vi "Trans_RT.vi"() -> ()   [LabVIEW 2016]
uses:
  PRIME Lab 2017b/Control/PRIME Control 2017b/Controls/GP307 cluster.ctl
  <vilib>/FPGAPlugInAG/cRIO-9067/niLvFpga_Open_cRIO-9067.vi
  <vilib>/Utility/error.llb/Error Cluster From Error Code.vi
  <vilib>/rvi/errors/niLvFpgaAdjustHostInterfaceError.vi
  <vilib>/functionblocks/Control/PID/PID.vi
  <vilib>/rvi/interface/nirviOpenFPGA/nirviOpenFPGA.xnode
  Builds/cRIOs/Trans-cRIO/FPGA/PRIMEControl2017_FPGA-Trans_FPGATrans_z3cvJGH+foY.lvbitx
  Trans_FPGA.vi
  <vilib>/rvi/interface/nirviReadWriteControl/nirviReadWriteControl.xnode
  <vilib>/functionblocks/FB Core/FB Core.xnode
  <vilib>/functionblocks/FB Property/FB Overlay DBL.ctl
  <vilib>/functionblocks/NI_FunctionBlock Libraries.lvlib
  <vilib>/NI_Real-Time Target Support.lvlib
  NiFpgaLv.dll
panel:
  in  "Tab Control":T1(tab)
  in  "derivative time (Td, min) -analyzer":dbl=0.05
  in  "integral time (Ti, min) -analyzer":dbl=0.01
  in  "proportional gain (Kc) -analyzer":dbl=25.0
  out "Analyzer mag command string":string
  out "analyzer field read":dbl
  out "Analyzer mag command":u8[](array[numeric])
  out "Analyzer mag field read":u8[](array[numeric])
  out "Analyzer mag field set":dbl
  in  "output high - analyzer":dbl=300.0
  in  "output low - analyzer":dbl
  out "Switch mag field set":dbl
  out "Switch mag field read":u8[](array[numeric])
  out "switch mag field read":dbl
  out "Switch mag command":u8[](array[numeric])
  in  "derivative time (Td, min) - switch":dbl=0.01
  in  "integral time (Ti, min) - switch":dbl=0.01
  in  "proportional gain (Kc) - switch":dbl=10.0
  out "Switch mag command string":string
  in  "output high - switch":dbl=250.0
  in  "output low - switch":dbl
  out "ExB mag command":u8[](array[numeric])
  out "EXB mag current set":dbl
  out "ExB mag command string":string
  out "Switch Mag addr command":u8[](array[numeric])
  out "Switch Mag ps trig":u8[](array[numeric])
  out "Steerer X+":dbl
  out "Steerer X-":dbl
  out "Steerer Y+":dbl
  out "Steerer Y-":dbl
  out "ExB +":dbl
  out "ExB -":dbl
  out "X+ V":fxp<+/-,26,5> format="%.23g"
  out "X+ I":fxp<+/-,26,5> format="%_4g"
  out "X- V":fxp<+/-,26,5> format="%_4g"
  out "X- I":fxp<+/-,26,5> format="%_4g"
  out "Y+ V":fxp<+/-,26,5> format="%_4g"
  out "Y+ I":fxp<+/-,26,5> format="%_4g"
  out "Y- V":fxp<+/-,26,5> format="%_4g"
  out "Y- I":fxp<+/-,26,5> format="%_4g"
  out "ExB+ V":fxp<+/-,26,5> format="%_4g"
  out "ExB+ I":fxp<+/-,26,5> format="%_4g"
  out "ExB- V":fxp<+/-,26,5> format="%_4g"
  out "ExB- I":fxp<+/-,26,5> format="%_4g"
  in  "Ion gauge cluster control":T2
  out "Analyze image vac gauge cluster":T3
  out "Switch object vac gauge cluster":T3
  out "Convectron 4":u8[](array[numeric])
  out "Ion gauge 4":u8[](array[numeric])
  out "Convectron 3":u8[](array[numeric])
  out "Ion gauge 3":u8[](array[numeric])
  out "Convectron 2":u8[](array[numeric])
  out "Ion gauge 2":u8[](array[numeric])
  out "Convectron 1":u8[](array[numeric])
  out "Ion gauge 1":u8[](array[numeric])
  out "Readback loop error":errorcluster
  out "Vacuum loop error":errorcluster
  out "Control Loop error":errorcluster
  out "ExB error":errorcluster
  out "Switch Magnet error":errorcluster
  out "Analyzer Magnet error":errorcluster
  out "Trans RT Error":errorcluster
  out "Trans FPGA error":errorcluster
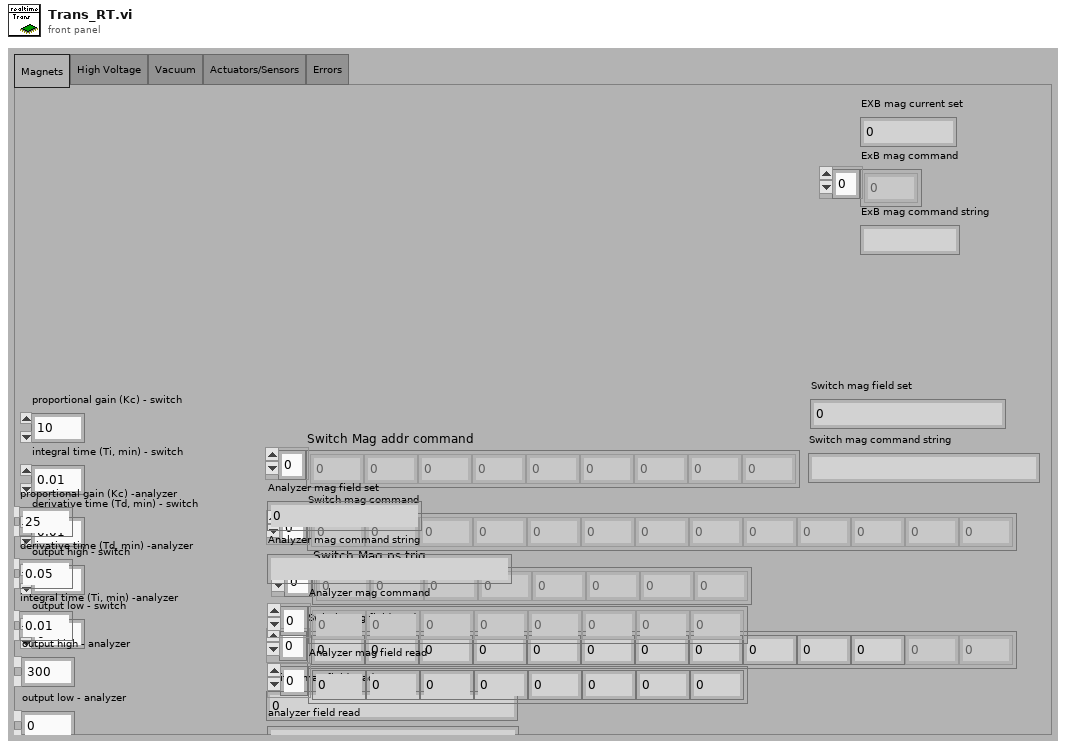
[diagram p1: front panel]
types:
  T1 = enum32{"Magnets", "High Voltage", "Vacuum", "Actuators/Sensors", "Errors"}
  T2 = typedef "GP307 cluster.ctl" = cluster{"Ion gauge 1":string, "Convectron  Gauge 1 ":string, "Ion Gauge 2":string, "Convectrom Gauge 2":string}
  T3 = cluster{"Ion gauge 1":string, "Convectron  Gauge 1 ":string, "Ion Gauge 2":string, "Convectrom Gauge 2":string}
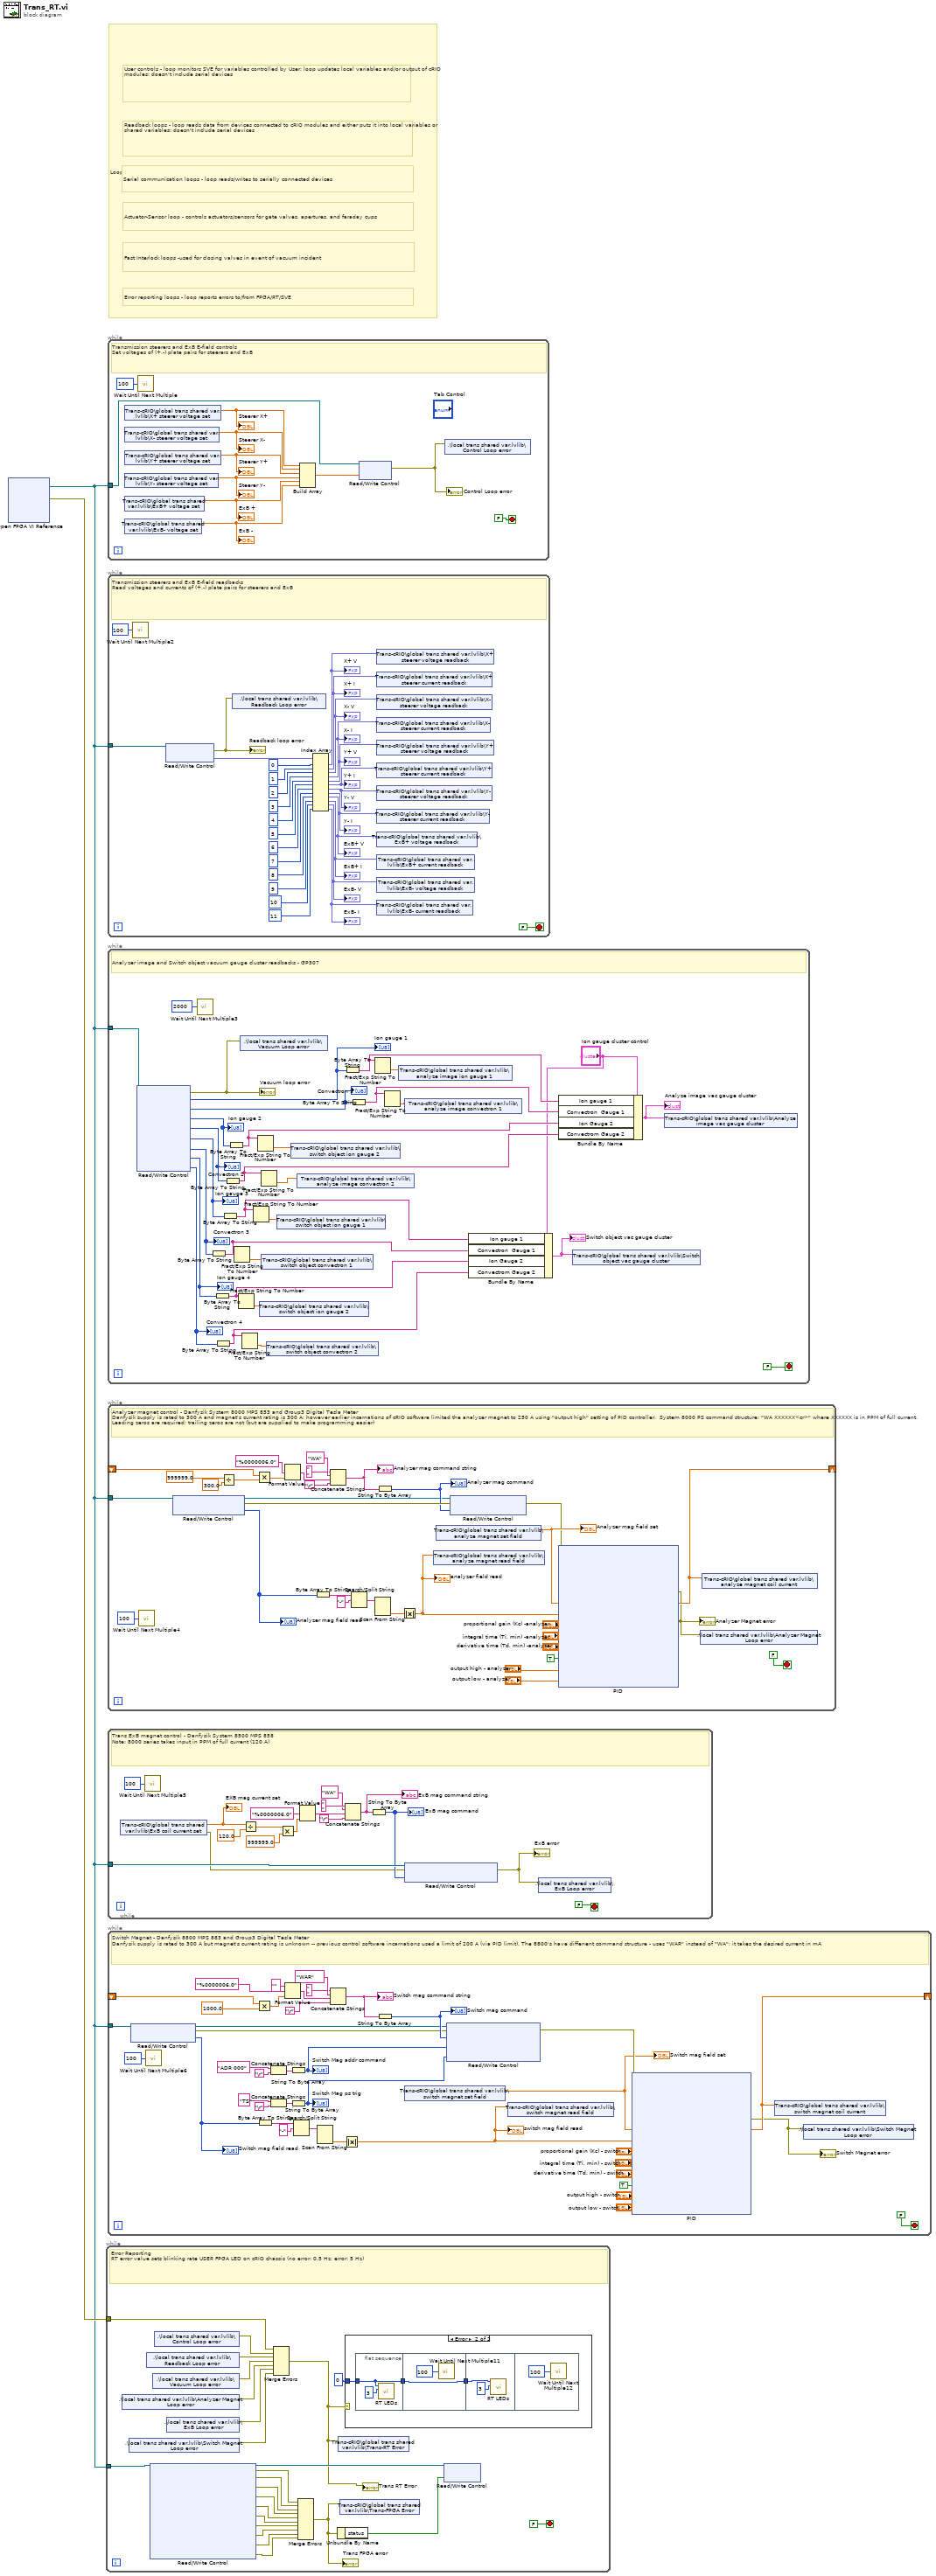
[diagram p0: block diagram]
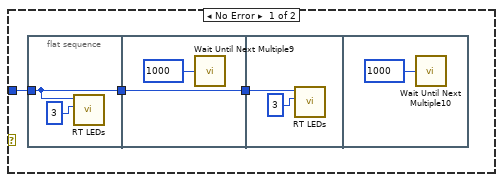
[diagram p2: hidden frame]
diagram:
  # "Serial communication loops - loop reads/writes to serially connected devices"
  # "Actuator-Sensor loop - controls actuators/sensors for gate valves, apertures, and faraday cups"
  # "Fast Interlock loops -used for closing valves in event of vacuum incident"
  # "Error reporting loops - loop reports errors to/from FPGA/RT/SVE"
  # "Readback loops - loop reads data from devices connected to cRIO modules and either puts it into local variables or shared variables; doesn't include serial devices"
  # "User controls - loop monitors SVE for variables controlled by User; loop updates local variables and/or output of cRIO modules; doesn't include serial devices"
  # "Loop legend - loops are color coded by responsibility"
  n1 = xnode "Open FPGA VI Reference"() -> ("FPGA VI Reference Out"=w1:refnum<k20>, "error out"=w2:errorcluster)  [unwired: 2 in]
  n2 = while {
    tunnel: w1 -> [w25]
    tunnel: w2 -> [w4]
    stop <- FALSE stop-if-true
    # "Error Reporting\nRT error value sets blinking rate USER FPGA LED on cRIO chassis (no error: 0.5 Hz; error: 5 Hz)"
    n3 = shared-variable ".\\local trans shared var.lvlib\\Analyzer Magnet Loop error"() -> (w10:errorcluster)  [unwired: 1 in, 1 out]
    n4 = shared-variable ".\\local trans shared var.lvlib\\Switch Magnet Loop error"() -> (w12:errorcluster)  [unwired: 1 in, 1 out]
    n5 = shared-variable ".\\local trans shared var.lvlib\\Readback Loop error"() -> (w8:errorcluster)  [unwired: 1 in, 1 out]
    n6 = xnode "Read/Write Control"("FPGA VI Reference In"=w25) -> ("FPGA VI Reference Out"=w24:refnum<k20>, "error out"=w13:errorcluster, "9205 error"=w23:errorcluster, "9264 error"=w22:errorcluster, "Analyzer PS error"=w21:errorcluster, "ExB PS error"=w20:errorcluster, "Switch PS error"=w19:errorcluster, "Analyzer Hall Probe error"=w18:errorcluster, "Switch Hall Probe error"=w17:errorcluster, "Analyze Image Vacuum Error"=w16:errorcluster, "Switch Object Vacuum Error"=w15:errorcluster)  [unwired: 1 in]
    n7 = shared-variable ".\\local trans shared var.lvlib\\Vacuum Loop error"() -> (w9:errorcluster)  [unwired: 1 in, 1 out]
    n8 = shared-variable ".\\local trans shared var.lvlib\\Control Loop error"() -> (w7:errorcluster)  [unwired: 1 in, 1 out]
    n9 = shared-variable ".\\local trans shared var.lvlib\\ExB Loop error"() -> (w11:errorcluster)  [unwired: 1 in, 1 out]
    n10 = Merge Errors(w4, w7, w8, w9, w10, w11, w12) -> (w3:errorcluster)
    "Trans RT Error" <- w3
    n11 = Merge Errors(w13, w23, w22, w21, w20, w19, w18, w17, w16, w15) -> (w6:errorcluster)
    "Trans FPGA error" <- w6
    n12 = Unbundle By Name(w6) -> ("status"=w26:bool)
    n13 = shared-variable "Trans-cRIO\\global trans shared var.lvlib\\Trans-RT Error"(w3) -> ()  [unwired: 1 in, 1 out]
    n14 = shared-variable "Trans-cRIO\\global trans shared var.lvlib\\Trans-FPGA Error"(w6) -> ()  [unwired: 1 in, 1 out]
    n15 = case shown="Error" w3 {
      tunnel: 0 -> [w29 w37]
      frame No Error {
        n16 = flat-sequence {
          tunnel: w29 -> [w30]
          tunnel: [w30] -> w27
          tunnel: [w32] -> w28
          tunnel: w27 -> [w32]
          tunnel: w28 -> [w34]
          frame #0 {
            n17 = call <vilib>:"RT LEDs.vi"("State"=3, "LED Num"=w30) -> ()  [unwired: 4 in, 2 out]
          }
          frame #1 {
            n18 = call "Wait Until Next Multiple9"("Count(mSec)"=u16 1000) -> ()  [unwired: 1 out]
          }
          frame #2 {
            n19 = call <vilib>:"RT LEDs.vi"("State"=3, "LED Num"=w34) -> ()  [unwired: 4 in, 2 out]
          }
          frame #3 {
            n20 = call "Wait Until Next Multiple10"("Count(mSec)"=u16 1000) -> ()  [unwired: 1 out]
          }
        }
      }
      frame Error {
        n21 = flat-sequence {
          tunnel: [w40] -> w39
          tunnel: w37 -> [w40]
          tunnel: w39 -> [w42]
          tunnel: [w42] -> w38
          tunnel: w38 -> [w44]
          frame #0 {
            n22 = call <vilib>:"RT LEDs.vi"("State"=3, "LED Num"=w40) -> ()  [unwired: 4 in, 2 out]
          }
          frame #1 {
            n23 = call "Wait Until Next Multiple11"("Count(mSec)"=u16 100) -> ()  [unwired: 1 out]
          }
          frame #2 {
            n24 = call <vilib>:"RT LEDs.vi"("State"=3, "LED Num"=w44) -> ()  [unwired: 4 in, 2 out]
          }
          frame #3 {
            n25 = call "Wait Until Next Multiple12"("Count(mSec)"=u16 100) -> ()  [unwired: 1 out]
          }
        }
      }
    }
    n26 = xnode "Read/Write Control"("FPGA VI Reference In"=w24, "RT error"=w26) -> ()  [unwired: 1 in, 2 out]
  }
  n27 = while {
    tunnel: w1 -> [w48]
    stop <- FALSE stop-if-true
    # "Transmission steerers and ExB E-field controls\nSet voltages of (+,-) plate pairs for steerers and ExB"
    n28 = shared-variable "Trans-cRIO\\global trans shared var.lvlib\\X+ steerer voltage set"() -> (w50:dbl)  [unwired: 1 in, 1 out]
    "Steerer X+" <- w50
    n29 = shared-variable "Trans-cRIO\\global trans shared var.lvlib\\X- steerer voltage set"() -> (w51:dbl)  [unwired: 1 in, 1 out]
    "Steerer X-" <- w51
    n30 = shared-variable "Trans-cRIO\\global trans shared var.lvlib\\Y+ steerer voltage set"() -> (w52:dbl)  [unwired: 1 in, 1 out]
    "Steerer Y+" <- w52
    n31 = shared-variable "Trans-cRIO\\global trans shared var.lvlib\\Y- steerer voltage set"() -> (w53:dbl)  [unwired: 1 in, 1 out]
    "Steerer Y-" <- w53
    n32 = shared-variable "Trans-cRIO\\global trans shared var.lvlib\\ExB+ voltage set"() -> (w54:dbl)  [unwired: 1 in, 1 out]
    "ExB +" <- w54
    n33 = shared-variable "Trans-cRIO\\global trans shared var.lvlib\\ExB- voltage set"() -> (w55:dbl)  [unwired: 1 in, 1 out]
    "ExB -" <- w55
    n34 = call "Wait Until Next Multiple"("Count(mSec)"=u32 100 ("millisecond multiple")) -> ()  [unwired: 1 out]
    n35 = Build Array(w50, w51, w52, w53, w54, w55) -> (w57:dbl[])
    n36 = xnode "Read/Write Control"("FPGA VI Reference In"=w48, "HV Set"=w57) -> ("error out"=w49:errorcluster)  [unwired: 1 in, 1 out]
    "Control Loop error" <- w49
    n37 = shared-variable ".\\local trans shared var.lvlib\\Control Loop error"(w49) -> ()  [unwired: 1 in, 1 out]
  }
  n38 = while {
    tunnel: w1 -> [w60]
    stop <- FALSE stop-if-true
    # "Transmission steerers and ExB E-field readbacks\nRead voltages and currents of (+,-) plate pairs for steerers and ExB"
    n39 = call "Wait Until Next Multiple2"("Count(mSec)"=u32 100 ("millisecond multiple")) -> ()  [unwired: 1 out]
    n40 = xnode "Read/Write Control"("FPGA VI Reference In"=w60) -> ("error out"=w59:errorcluster, "HV monitor"=w86:fxp<+/-,26,5>[])  [unwired: 1 in, 1 out]
    "Readback loop error" <- w59
    n41 = shared-variable ".\\local trans shared var.lvlib\\Readback Loop error"(w59) -> ()  [unwired: 1 in, 1 out]
    n42 = Index Array(array=w86, index #1=0 ("index"), index #2=1 ("index"), index #3=2 ("index"), index #4=3 ("index"), index #5=4 ("index"), index #6=5 ("index"), index #7=6 ("index"), index #8=7 ("index"), index #9=8 ("index"), index #10=9 ("index"), index #11=10 ("index"), index #12=11 ("index")) -> (element #1=w75:fxp<+/-,26,5>, element #2=w77:fxp<+/-,26,5>, element #3=w76:fxp<+/-,26,5>, element #4=w74:fxp<+/-,26,5>, element #5=w78:fxp<+/-,26,5>, element #6=w80:fxp<+/-,26,5>, element #7=w79:fxp<+/-,26,5>, element #8=w81:fxp<+/-,26,5>, element #9=w82:fxp<+/-,26,5>, element #10=w84:fxp<+/-,26,5>, element #11=w83:fxp<+/-,26,5>, element #12=w85:fxp<+/-,26,5>)
    "X+ V" <- w75
    "X+ I" <- w77
    "X- V" <- w76
    "X- I" <- w74
    "Y+ V" <- w78
    "Y+ I" <- w80
    "Y- V" <- w79
    "Y- I" <- w81
    "ExB+ V" <- w82
    "ExB+ I" <- w84
    "ExB- V" <- w83
    "ExB- I" <- w85
    n43 = shared-variable "Trans-cRIO\\global trans shared var.lvlib\\X+ steerer voltage readback"(w75) -> ()  [unwired: 1 in, 1 out]
    n44 = shared-variable "Trans-cRIO\\global trans shared var.lvlib\\X+ steerer current readback"(w77) -> ()  [unwired: 1 in, 1 out]
    n45 = shared-variable "Trans-cRIO\\global trans shared var.lvlib\\X- steerer voltage readback"(w76) -> ()  [unwired: 1 in, 1 out]
    n46 = shared-variable "Trans-cRIO\\global trans shared var.lvlib\\X- steerer current readback"(w74) -> ()  [unwired: 1 in, 1 out]
    n47 = shared-variable "Trans-cRIO\\global trans shared var.lvlib\\Y+ steerer voltage readback"(w78) -> ()  [unwired: 1 in, 1 out]
    n48 = shared-variable "Trans-cRIO\\global trans shared var.lvlib\\Y+ steerer current readback"(w80) -> ()  [unwired: 1 in, 1 out]
    n49 = shared-variable "Trans-cRIO\\global trans shared var.lvlib\\Y- steerer voltage readback"(w79) -> ()  [unwired: 1 in, 1 out]
    n50 = shared-variable "Trans-cRIO\\global trans shared var.lvlib\\Y- steerer current readback"(w81) -> ()  [unwired: 1 in, 1 out]
    n51 = shared-variable "Trans-cRIO\\global trans shared var.lvlib\\ExB+ voltage readback"(w82) -> ()  [unwired: 1 in, 1 out]
    n52 = shared-variable "Trans-cRIO\\global trans shared var.lvlib\\ExB+ current readback"(w84) -> ()  [unwired: 1 in, 1 out]
    n53 = shared-variable "Trans-cRIO\\global trans shared var.lvlib\\ExB- voltage readback"(w83) -> ()  [unwired: 1 in, 1 out]
    n54 = shared-variable "Trans-cRIO\\global trans shared var.lvlib\\ExB- current readback"(w85) -> ()  [unwired: 1 in, 1 out]
  }
  n55 = while {
    tunnel: w1 -> [w93]
    stop <- FALSE stop-if-true
    # "Analyzer image and Switch object vacuum gauge cluster readbacks - GP307"
    n56 = xnode "Read/Write Control"("FPGA VI Reference In"=w93) -> ("error out"=w92:errorcluster, "Ion gauge 1"=w114:u8[], "Convectron 1"=w115:u8[], "Ion gauge 2"=w116:u8[], "Convectron 2"=w117:u8[], "Ion gauge 3"=w112:u8[], "Convectron 3"=w111:u8[], "Ion gauge 4"=w90:u8[], "Convectron 4"=w89:u8[])  [unwired: 1 in, 1 out]
    "Vacuum loop error" <- w92
    "Ion gauge 1" <- w114
    "Convectron 1" <- w115
    "Ion gauge 2" <- w116
    "Convectron 2" <- w117
    "Ion gauge 3" <- w112
    "Convectron 3" <- w111
    "Ion gauge 4" <- w90
    "Convectron 4" <- w89
    n57 = call "Wait Until Next Multiple3"("Count(mSec)"=u32 2000 ("millisecond multiple")) -> ()  [unwired: 1 out]
    n58 = Byte Array To String(unsigned byte array=w111) -> (string=w108:string)
    n59 = Byte Array To String(unsigned byte array=w90) -> (string=w107:string)
    n60 = Byte Array To String(unsigned byte array=w89) -> (string=w106:string)
    n61 = Byte Array To String(unsigned byte array=w112) -> (string=w109:string)
    n62 = Byte Array To String(unsigned byte array=w117) -> (string=w99:string)
    n63 = Byte Array To String(unsigned byte array=w116) -> (string=w98:string)
    n64 = Fract/Exp String To Number(string=w108) -> (number=w104:dbl)  [unwired: 3 in, 1 out]
    n65 = Fract/Exp String To Number(string=w107) -> (number=w103:dbl)  [unwired: 3 in, 1 out]
    n66 = shared-variable ".\\local trans shared var.lvlib\\Vacuum Loop error"(w92) -> ()  [unwired: 1 in, 1 out]
    n67 = Fract/Exp String To Number(string=w106) -> (number=w102:dbl)  [unwired: 3 in, 1 out]
    n68 = Fract/Exp String To Number(string=w109) -> (number=w105:dbl)  [unwired: 3 in, 1 out]
    n69 = Fract/Exp String To Number(string=w98) -> (number=w96:dbl)  [unwired: 3 in, 1 out]
    n70 = shared-variable "Trans-cRIO\\global trans shared var.lvlib\\switch object ion gauge 2"(w103) -> ()  [unwired: 1 in, 1 out]
    n71 = Fract/Exp String To Number(string=w99) -> (number=w94:dbl)  [unwired: 3 in, 1 out]
    n72 = shared-variable "Trans-cRIO\\global trans shared var.lvlib\\switch object convectron 1"(w104) -> ()  [unwired: 1 in, 1 out]
    n73 = shared-variable "Trans-cRIO\\global trans shared var.lvlib\\switch object convectron 2"(w102) -> ()  [unwired: 1 in, 1 out]
    n74 = shared-variable "Trans-cRIO\\global trans shared var.lvlib\\switch object ion gauge 1"(w105) -> ()  [unwired: 1 in, 1 out]
    n75 = shared-variable "Trans-cRIO\\global trans shared var.lvlib\\switch object ion gauge 2"(w96) -> ()  [unwired: 1 in, 1 out]
    n76 = shared-variable "Trans-cRIO\\global trans shared var.lvlib\\analyze image convectron 2"(w94) -> ()  [unwired: 1 in, 1 out]
    n77 = Byte Array To String(unsigned byte array=w114) -> (string=w101:string)
    n78 = Byte Array To String(unsigned byte array=w115) -> (string=w100:string)
    n79 = Fract/Exp String To Number(string=w101) -> (number=w97:dbl)  [unwired: 3 in, 1 out]
    n80 = Fract/Exp String To Number(string=w100) -> (number=w95:dbl)  [unwired: 3 in, 1 out]
    n81 = shared-variable "Trans-cRIO\\global trans shared var.lvlib\\analyze image ion gauge 1"(w97) -> ()  [unwired: 1 in, 1 out]
    n82 = shared-variable "Trans-cRIO\\global trans shared var.lvlib\\analyze image convectron 1"(w95) -> ()  [unwired: 1 in, 1 out]
    n83 = Bundle By Name(cluster="Ion gauge cluster control", "Ion gauge 1"=w109, "Convectron  Gauge 1"=w108, "Ion Gauge 2"=w107, "Convectrom Gauge 2"=w106) -> (w110:T2)
    "Switch object vac gauge cluster" <- w110
    n84 = Bundle By Name(cluster="Ion gauge cluster control", "Ion gauge 1"=w101, "Convectron  Gauge 1"=w100, "Ion Gauge 2"=w98, "Convectrom Gauge 2"=w99) -> (w91:T2)
    "Analyze image vac gauge cluster" <- w91
    n85 = shared-variable "Trans-cRIO\\global trans shared var.lvlib\\Switch object vac gauge cluster"(w110) -> ()  [unwired: 1 in, 1 out]
    n86 = shared-variable "Trans-cRIO\\global trans shared var.lvlib\\Analyze image vac gauge cluster"(w91) -> ()  [unwired: 1 in, 1 out]
  }
  n87 = while {
    shift-right: [w136] -> _
    shift-left: _ -> [w127]
    tunnel: w1 -> [w131]
    stop <- FALSE stop-if-true
    # "Analyzer magnet control - Danfysik System 8000 MPS 853 and Group3 Digital Tesla Meter\nDanfysik supply is rated to 300 A and magnet's current rating is 300 A; however earlier incarnations of cRIO software limited the analyzer magnet to 250 A using \"output high\" setting of PID controller.  System 8000 PS command structure: \"WA XXXXXX<cr>\" where XXXXXX is in PPM of full current. Leading zeros are required; trailing zeros are not (but are supplied to make programming easier)"
    n88 = call "Wait Until Next Multiple4"("Count(mSec)"=u32 100 ("millisecond multiple")) -> ()  [unwired: 1 out]
    n89 = xnode "Read/Write Control"("FPGA VI Reference In"=w131) -> ("FPGA VI Reference Out"=w123:refnum<k20>, "error out"=w130:errorcluster, "analyzer mag field"=w126:u8[])  [unwired: 1 in]
    "Analyzer mag field read" <- w126
    n90 = Divide(x=999999.0, y=300.0) -> (x/y=w143:dbl)
    n91 = Multiply(x=w127, y=w143) -> (x*y=w145:dbl)
    n92 = Format Value(format string="%0000006.0", value (0)=w145) -> (output string=w148:string)  [unwired: 1 out]
    n93 = Byte Array To String(unsigned byte array=w126) -> (string=w138:string)
    n94 = Concatenate Strings("WA", " ", w148, "\r") -> (w149:string)
    "Analyzer mag command string" <- w149
    n95 = Search/Split String(string=w138, search string/char (-)="-") -> (match + rest of string=w128:string)  [unwired: 3 out]
    n96 = Scan From String(input string=w128) -> (output 1=w137:dbl)  [unwired: 3 in, 4 out]
    n97 = String To Byte Array(string=w149) -> (unsigned byte array=w129:u8[])
    "Analyzer mag command" <- w129
    n98 = Absolute Value(x=w137) -> (abs(x)=w124:dbl)
    "analyzer field read" <- w124
    n99 = shared-variable "Trans-cRIO\\global trans shared var.lvlib\\analyze magnet read field"(w124) -> ()  [unwired: 1 in, 1 out]
    n100 = shared-variable "Trans-cRIO\\global trans shared var.lvlib\\analyze magnet set field"() -> (w125:dbl)  [unwired: 1 in, 1 out]
    "Analyzer mag field set" <- w125
    n101 = xnode "Read/Write Control"("FPGA VI Reference In"=w123, "error in"=w130, "analyzer mag ps set"=w129) -> ("error out"=w122:errorcluster)  [unwired: 1 out]
    n102 = xnode "PID"("error in"=w122, "setpoint"=w125, "process variable"=w124, "proportional gain (Kc)"="proportional gain (Kc) -analyzer", "integral time (Ti, min)"="integral time (Ti, min) -analyzer", "derivative time (Td, min)"="derivative time (Td, min) -analyzer", "auto? (T)"=TRUE, "output high"="output high - analyzer", "output low"="output low - analyzer") -> ("error out"=w121:errorcluster, "output"=w136:dbl)
    "Analyzer Magnet error" <- w121
    n103 = shared-variable ".\\local trans shared var.lvlib\\Analyzer Magnet Loop error"(w121) -> ()  [unwired: 1 in, 1 out]
    n104 = shared-variable "Trans-cRIO\\global trans shared var.lvlib\\analyze magnet coil current"(w136) -> ()  [unwired: 1 in, 1 out]
  }
  n105 = while {
    tunnel: w1 -> [w226]
    stop <- FALSE stop-if-true
    # "Trans ExB magnet control - Danfysik System 8500 MPS 858\nNote: 8000 series takes input in PPM of full current (120 A)"
    n106 = shared-variable "Trans-cRIO\\global trans shared var.lvlib\\ExB coil current set"() -> (w219:dbl, error out=w223:errorcluster)  [unwired: 1 in]
    "EXB mag current set" <- w219
    n107 = call "Wait Until Next Multiple5"("Count(mSec)"=u32 100 ("millisecond multiple")) -> ()  [unwired: 1 out]
    n108 = Divide(x=w219, y=120.0) -> (x/y=w218:dbl)
    n109 = Multiply(x=w218, y=999999.0 ("x")) -> (x*y=w220:dbl)
    n110 = Format Value(format string="%0000006.0", value (0)=w220) -> (output string=w230:string)  [unwired: 1 out]
    n111 = Concatenate Strings("WA", " ", w230, "\r") -> (w227:string)
    "ExB mag command string" <- w227
    n112 = String To Byte Array(string=w227) -> (unsigned byte array=w224:u8[])
    "ExB mag command" <- w224
    n113 = xnode "Read/Write Control"("FPGA VI Reference In"=w226, "error in"=w223, "trans ExB mag ps set"=w224) -> ("error out"=w225:errorcluster)  [unwired: 1 out]
    "ExB error" <- w225
    n114 = shared-variable ".\\local trans shared var.lvlib\\ExB Loop error"(w225) -> ()  [unwired: 1 in, 1 out]
  }
  n115 = while {
    shift-right: [w263] -> _
    shift-left: _ -> [w257]
    tunnel: w1 -> [w244]
    stop <- FALSE stop-if-true
    # "Switch Magnet - Danfysik 8800 MPS 883 and Group3 Digital Tesla Meter\nDanfysik supply is rated to 300 A but magnet's current rating is unknown -- previous control software incarnations used a limit of 200 A (via PID limit). The 8800's have diffenent command structure - uses \"WAR\" instead of \"WA\"; it takes the desired current in mA"
    n116 = xnode "Read/Write Control"("FPGA VI Reference In"=w244) -> ("FPGA VI Reference Out"=w241:refnum<k20>, "error out"=w240:errorcluster, "switch mag field"=w256:u8[])  [unwired: 1 in]
    "Switch mag field read" <- w256
    n117 = call "Wait Until Next Multiple6"("Count(mSec)"=u32 100 ("millisecond multiple")) -> ()  [unwired: 1 out]
    n118 = Multiply(x=w257, y=1000.0) -> (x*y=w269:dbl)
    n119 = Byte Array To String(unsigned byte array=w256) -> (string=w265:string)
    n120 = Concatenate Strings("ADR 000" ("Write String"), "\r") -> (w245:string)
    n121 = Concatenate Strings("TS" ("Write String"), "\r") -> (w236:string)
    n122 = Format Value(string ("")="", format string="%0000006.0", value (0)=w269) -> (output string=w272:string)
    n123 = String To Byte Array(string=w245) -> (unsigned byte array=w243:u8[])
    "Switch Mag addr command" <- w243
    n124 = String To Byte Array(string=w236) -> (unsigned byte array=w235:u8[])
    "Switch Mag ps trig" <- w235
    n125 = Search/Split String(string=w265, search string/char (-)="-") -> (match + rest of string=w258:string)  [unwired: 3 out]
    n126 = Scan From String(input string=w258) -> (output 1=w264:dbl)  [unwired: 3 in, 4 out]
    n127 = Concatenate Strings("WAR", " ", w272, "\r") -> (w273:string)
    "Switch mag command string" <- w273
    n128 = Absolute Value(x=w264) -> (abs(x)=w255:dbl)
    "switch mag field read" <- w255
    n129 = String To Byte Array(string=w273) -> (unsigned byte array=w242:u8[])
    "Switch mag command" <- w242
    n130 = shared-variable "Trans-cRIO\\global trans shared var.lvlib\\switch magnet set field"() -> (w234:dbl)  [unwired: 1 in, 1 out]
    "Switch mag field set" <- w234
    n131 = xnode "Read/Write Control"("FPGA VI Reference In"=w241, "error in"=w240, "switch mag ps set"=w242, "Switch Mag addr"=w243, "switch mag ps trig"=w235) -> ("error out"=w239:errorcluster)  [unwired: 1 out]
    n132 = shared-variable "Trans-cRIO\\global trans shared var.lvlib\\switch magnet read field"(w255) -> ()  [unwired: 1 in, 1 out]
    n133 = xnode "PID"("error in"=w239, "setpoint"=w234, "process variable"=w255, "proportional gain (Kc)"="proportional gain (Kc) - switch", "integral time (Ti, min)"="integral time (Ti, min) - switch", "derivative time (Td, min)"="derivative time (Td, min) - switch", "auto? (T)"=TRUE, "output high"="output high - switch", "output low"="output low - switch") -> ("error out"=w254:errorcluster, "output"=w263:dbl)
    "Switch Magnet error" <- w254
    n134 = shared-variable "Trans-cRIO\\global trans shared var.lvlib\\switch magnet coil current"(w263) -> ()  [unwired: 1 in, 1 out]
    n135 = shared-variable ".\\local trans shared var.lvlib\\Switch Magnet Loop error"(w254) -> ()  [unwired: 1 in, 1 out]
  }
